vi "plot_boat.vi"(4 "Rudder Setpoint":T3 min=-0.95 max=0.95 scale=1.0..-1.0, 6 "Sail Setpoints":T4 {"MainSailSuggestion" min=0.0 max=1.0; "JibSailSuggestion" min=0.0 max=1.0}, 7 "Trace Path":bool=TRUE, 8 "Heading":dbl, 9 "MapDistanceInfo":T1 {"Top Left Pixel UTM"."North" format="%#_10f"; "Top Left Pixel UTM"."East" format="%#_8f"; "Bottom Right Pixel UTM"."North" format="%#_10f"; "Bottom Right Pixel UTM"."East" format="%#_8f"}, 10 "UTM Location":T2 {"North" format="%#_10f"; "East" format="%#_8f"}, 11 "Map in":T5) -> (1 "MapDistanceInfo OUT":T1 {"Top Left Pixel UTM"."North" format="%#_10f"; "Top Left Pixel UTM"."East" format="%#_8f"; "Bottom Right Pixel UTM"."North" format="%#_10f"; "Bottom Right Pixel UTM"."East" format="%#_8f"}, 2 "Boat Outside Img":bool, 3 "Map Out":T5)   [LabVIEW 2013]
uses:
  <vilib>/vision/Image Controls.llb/IMAQ Image.ctl
  cRIO_Code/Data/TypeDefs/UTM Location.ctl
  TypeDef/map_metadata.ctl
  cRIO_Code/Data/TypeDefs/Sail Set Suggestions.ctl
  cRIO_Code/Data/TypeDefs/Rudder Set Suggestions.ctl
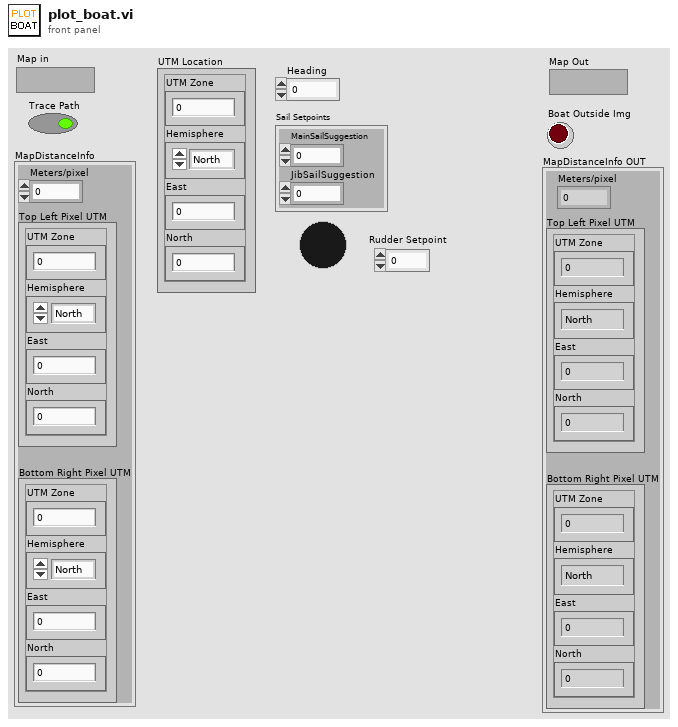
[diagram p1: front panel]
types:
  T1 = typedef "map_metadata.ctl" = cluster{"Meters/pixel":dbl, "Top Left Pixel UTM":T2, "Bottom Right Pixel UTM":T2}
  T2 = typedef "UTM Location.ctl" = cluster{"UTM Zone":dbl, "Hemisphere":enum16{"North", "South"}, "East":dbl, "North":dbl}
  T3 = typedef "Rudder Set Suggestions.ctl" = dbl
  T4 = typedef "Sail Set Suggestions.ctl" = cluster{"MainSailSuggestion":dbl, "JibSailSuggestion":dbl}
  T5 = typedef "IMAQ Image.ctl" = refnum<image>
  T6 = typedef "boat_overlay_references.ctl" = cluster{"Boat Icon, Unrotated":T5, "Boat Icon, Rotated":T5, "Mainsail Icon, Unrotated":T5, "Mainsail Icon, Rotated":T5, "Jib Icon, Rotated":T5, "Jib Icon, Unrotated":T5, "Rudder Icon, Rotated":T5, "Rudder Icon, Unrotated":T5}
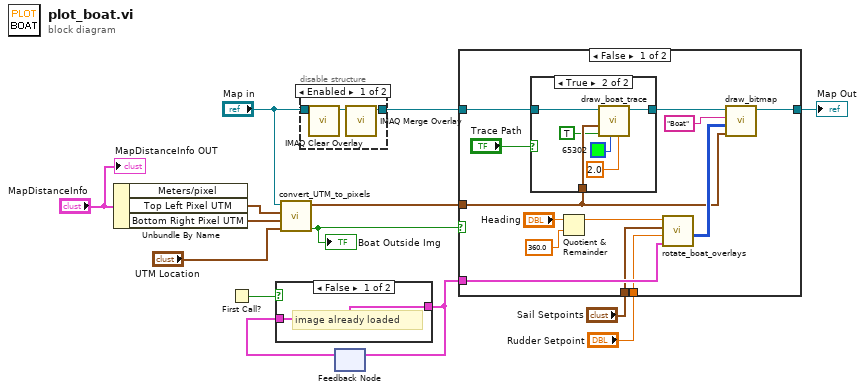
[diagram p0: block diagram]
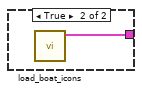
[diagram p5: hidden frame]
diagram:
  n1 = Unbundle By Name("MapDistanceInfo") -> ("Top Left Pixel UTM"=w6:T2, "Bottom Right Pixel UTM"=w5:T2)  [unwired: 1 out]
  n2 = First Call?() -> (First Call?: T/F=w2:bool)
  n3 = call "convert_UTM_to_pixels.vi"("UTM position of Boat"="UTM Location", "Bottom Right Pixel UTM"=w5, "Top Left Pixel UTM"=w6, "Map in"="Map in") -> ("Boat Outside Img"=w9:bool, "Position"=w8:cluster{"X":i32, "Y":i32})  [unwired: 6 in]
  "Boat Outside Img" <- w9
  n4 = disable-structure shown="Enabled" {
    disable-tunnel: [w16 w18] -> w13
    disable-tunnel: "Map in" -> [w15 w18]
    frame Enabled {
      n5 = call "IMAQ Clear Overlay"("Image"=w15) -> ("Image Out"=w17:T5)  [unwired: 2 in, 8 out]
      n6 = call "IMAQ Merge Overlay"("Image Src"=w17) -> ("Image Dst Out"=w16:T5)  [unwired: 4 in, 6 out]
    }
    frame Disabled {
    }
  }
  n7 = feedback #1() -> (w1:T6)  [unwired: 1 in]
  n8 = case shown="False" w2 {
    tunnel: [w19 w20] -> w14
    tunnel: w1 -> [w19 _]
    frame False {
      # "image already loaded"
    }
    frame True {
      n9 = call "load_boat_icons.vi"() -> ("Boat Overlay References Out"=w20:T6)  [unwired: 11 in]
    }
  }
  n10 = feedback-in #1(w14) -> ()
  n11 = case shown="False" w9 {
    tunnel: [w32 w41] -> w12
    tunnel: w13 -> [w30 w41]
    tunnel: w14 -> [w24 _]
    tunnel: w8 -> [w29 _]
    tunnel: "Sail Setpoints" -> [w23 _]
    tunnel: "Rudder Setpoint" -> [w22 _]
    frame False {
      n12 = case shown="True" "Trace Path" {
        tunnel: [w34 w39] -> w31
        tunnel: w30 -> [w34 w38]
        tunnel: w29 -> [_ w37]
        frame False {
        }
        frame True {
          n13 = call "draw_boat_trace.vi"("Radius (px)"=2.0, "circle color"=u32 65302, "Merge Overlay?"=TRUE, "Position"=w37, "Image In"=w38) -> ("Image Out"=w39:T5)  [unwired: 6 in]
        }
      }
      n14 = Quotient & Remainder(x="Heading", y=360.0) -> (x-y*floor(x/y)=w27:dbl)  [unwired: 1 out]
      n15 = call "rotate_boat_overlays.vi"("Overlay References In"=w24, "Rudder Setpoint"=w22, "Sail Setpoints"=w23, "Heading"=w27) -> ("Rotated Boat Icon Bitmap Out"=w33:u32[][])  [unwired: 6 in, 1 out]
      n16 = call "draw_bitmap.vi"("Position"=w29, "Boat Bitmap"=w33, "Group"="Boat", "Image In"=w31) -> ("Image Out"=w32:T5)  [unwired: 3 out]
    }
    frame True {
      # "don't draw\nif boat\noutside\nimage why not? lol"
    }
  }
  "Map Out" <- w12
  "MapDistanceInfo OUT" <- "MapDistanceInfo"
